vi "Read RequirementsMap.vi"(11 "RequirementsFile in":refnum<class "RequirementMap.lvclass">) -> (2 "Requirements":map{string, string}(c390), 3 "RequirementsFile out":refnum<class "RequirementMap.lvclass">)   [LabVIEW 2021, in "Bananas.lvlib" / "RequirementMap.lvclass"]
uses:
  RequirementMap.lvclass
  RequirementMap.lvclass/RequirementMap.ctl
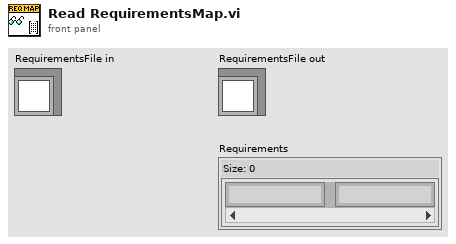
[diagram p1: front panel]
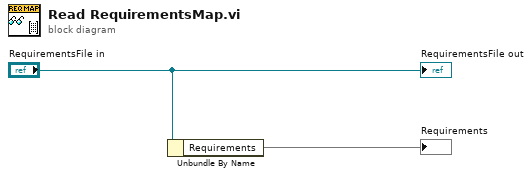
[diagram p0: block diagram]
diagram:
  n1 = Unbundle By Name("RequirementsFile in") -> ("Requirements"=→"Requirements":map{string, string})
  "RequirementsFile out" <- "RequirementsFile in"
